vi "ADCP_Get_Parameter_Instance.vi"(8 "error in (no error)":errorcluster, 9 "Parameter Index":i32=-1, 10 "Parameter name":string, 11 "ADCP in":refnum<class "ADCP.lvclass">) -> (0 "error out":errorcluster, 1 "Data Packet":T2, 2 "Parameter":T3, 3 "ADCP out":refnum<class "ADCP.lvclass">)   [LabVIEW 2017, in "ADCP.lvclass"]
uses:
  ADCP.lvclass
  ADCP_Data_Packet_Transmit_Mode.ctl
  ADCP.lvclass/ADCP.ctl
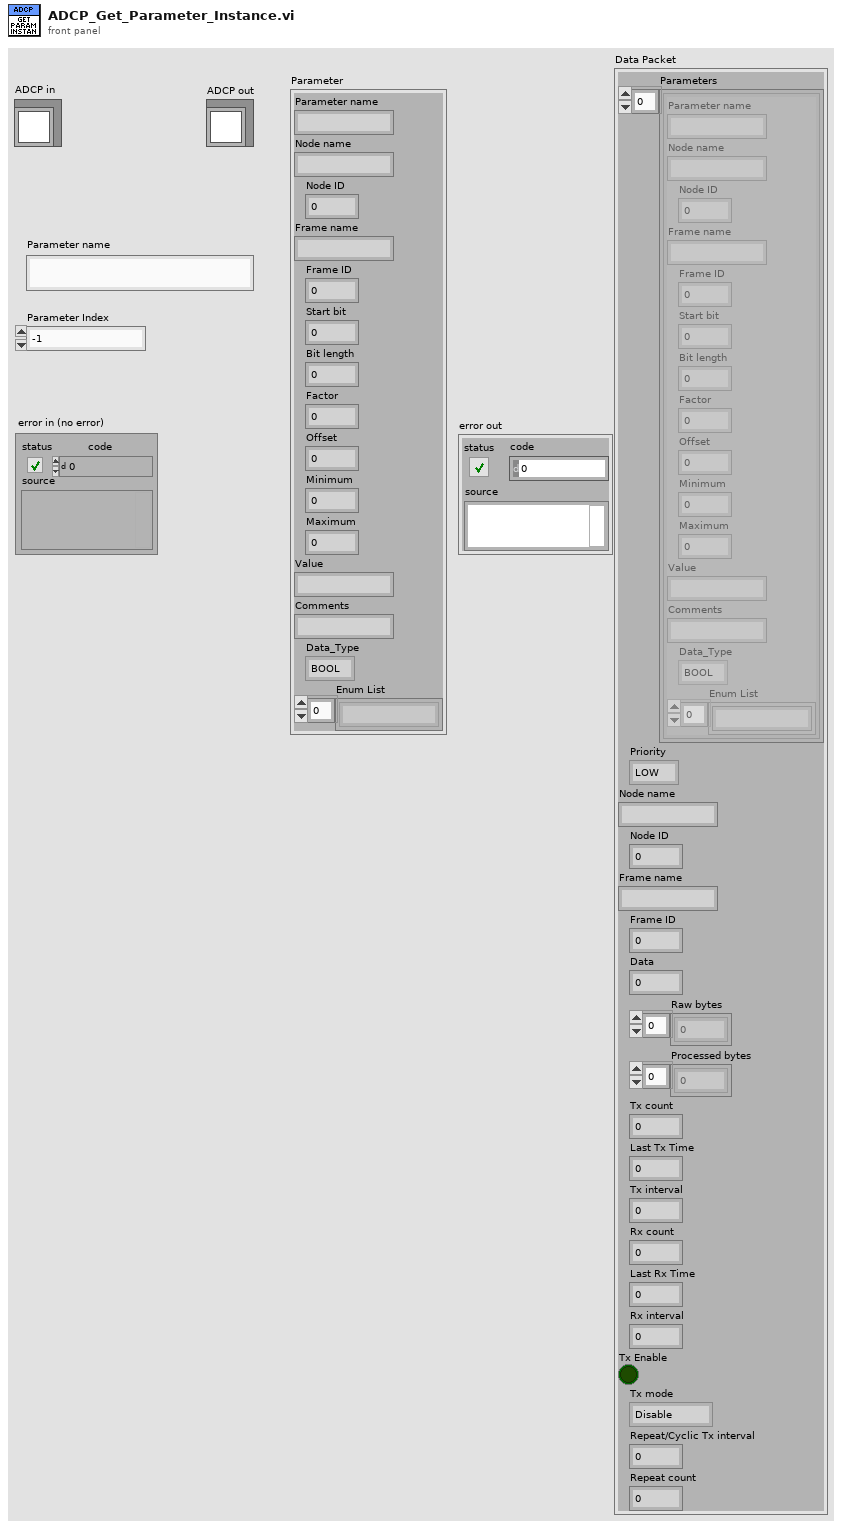
[diagram p1: front panel]
types:
  T1 = typedef "ADCP.lvclass/ADCP_Data_Packet_Transmit_Mode.ctl" = enum16{"Disable", "Single", "Cyclic", "Repeat"}
  T2 = cluster{"Parameters":cluster{"Parameter name":string, "Node name":string, "Node ID":u8, "Frame name":string, "Frame ID":u8, "Start bit":u32, "Bit length":u32, "Factor":dbl, "Offset":dbl, "Minimum":dbl, "Maximum":dbl, "Value":string, "Comments":string, "Data_Type":enum16{"BOOL", "UNSIGNED", "SIGNED", "FLOAT32", "ENUM"}, "Enum List":string[]}[], "Priority":enum16{"LOW", "HIGH"}, "Node name":string, "Node ID":u8, "Frame name":string, "Frame ID":u8, "Data":u32, "Raw bytes":u8[], "Processed bytes":u8[], "Tx count":i32, "Last Tx Time":u32, "Tx interval":u32, "Rx count":i32, "Last Rx Time":u32, "Rx interval":u32, "Tx Enable":bool, "Tx mode":T1, "Repeat/Cyclic Tx interval":u32, "Repeat count":u16}
  T3 = cluster{"Parameter name":string, "Node name":string, "Node ID":u8, "Frame name":string, "Frame ID":u8, "Start bit":u32, "Bit length":u32, "Factor":dbl, "Offset":dbl, "Minimum":dbl, "Maximum":dbl, "Value":string, "Comments":string, "Data_Type":enum16{"BOOL", "UNSIGNED", "SIGNED", "FLOAT32", "ENUM"}, "Enum List":string[]}
  T4 = cluster{"Parameter name":string, "Node name":string, "Node ID":u8, "Frame name":string, "Frame ID":u8, "Start bit":u32, "Bit length":u32, "Factor":dbl, "Offset":dbl, "Minimum":dbl, "Maximum":dbl, "Value":string, "Comments":string, "Data_Type":enum16{"BOOL", "UNSIGNED", "SIGNED", "FLOAT32", "ENUM"}, "Enum List":string[]}[]
  T5 = cluster{"Parameters":cluster{"Parameter name":string, "Node name":string, "Node ID":u8, "Frame name":string, "Frame ID":u8, "Start bit":u32, "Bit length":u32, "Factor":dbl, "Offset":dbl, "Minimum":dbl, "Maximum":dbl, "Value":string, "Comments":string, "Data_Type":enum16{"BOOL", "UNSIGNED", "SIGNED", "FLOAT32", "ENUM"}, "Enum List":string[]}[], "Priority":enum16{"LOW", "HIGH"}, "Node name":string, "Node ID":u8, "Frame name":string, "Frame ID":u8, "Data":u32, "Raw bytes":u8[], "Processed bytes":u8[], "Tx count":i32, "Last Tx Time":u32, "Tx interval":u32, "Rx count":i32, "Last Rx Time":u32, "Rx interval":u32, "Tx Enable":bool, "Tx mode":T1, "Repeat/Cyclic Tx interval":u32, "Repeat count":u16}[]
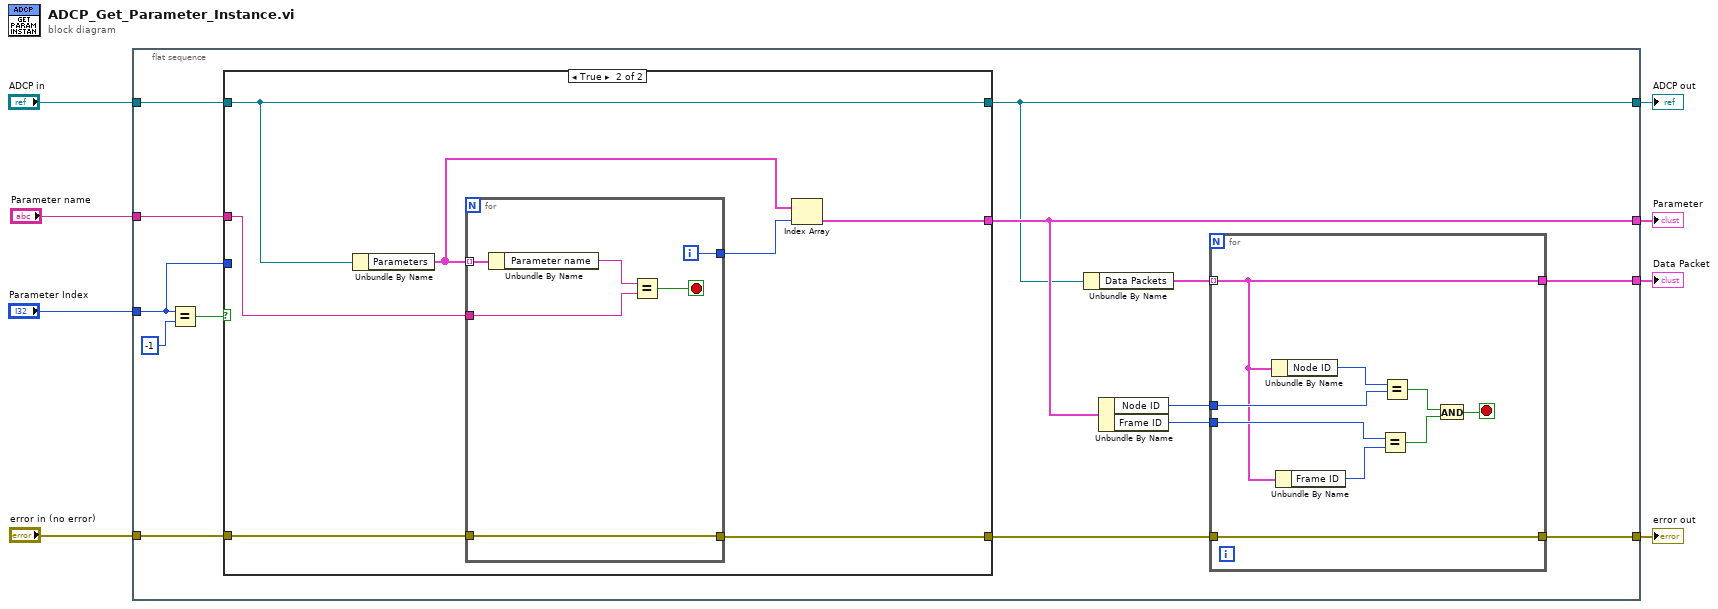
[diagram p0: block diagram]
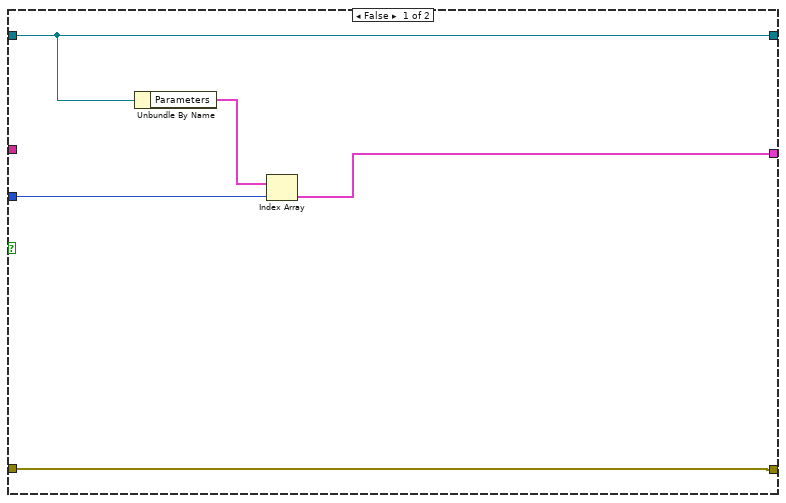
[diagram p2: hidden frame]
diagram:
  n1 = flat-sequence {
    tunnel: "ADCP in" -> [w19]
    tunnel: "Parameter name" -> [w18]
    tunnel: "Parameter Index" -> [w17]
    tunnel: "error in (no error)" -> [w22]
    tunnel: [w14] -> w4
    tunnel: [w11] -> w3
    tunnel: [w10] -> w2
    tunnel: [w9] -> w1
    frame #0 {
      n2 = Equal?(x=w17, y=-1) -> (x = y?=w21:bool)
      n3 = case shown="True" w21 {
        tunnel: w22 -> [w33 w43]
        tunnel: w19 -> [w32 w37]
        tunnel: w18 -> [_ w42]
        tunnel: w17 -> [w35 _]
        tunnel: [w34 w39] -> w14
        tunnel: [w33 w38] -> w16
        tunnel: [w32 w37] -> w9
        frame False {
          n4 = Unbundle By Name(w32) -> ("Parameters"=w36:T4)
          n5 = Index Array(array=w36, index=w35) -> (element=w34:T3)
        }
        frame True {
          n6 = Unbundle By Name(w37) -> ("Parameters"=w41:T4)
          n7 = for {
            tunnel: w41 -> [w49] mode=indexing
            tunnel: w43 -> [w45]
            tunnel: w42 -> [w47]
            tunnel: [w45] -> w38
            tunnel: [w44] -> w40
            i -> [w44]
            stop <- w46 stop-if-true
            n8 = Unbundle By Name(w49) -> ("Parameter name"=w48:string)
            n9 = Equal?(x=w48, y=w47) -> (x = y?=w46:bool)
          }
          n10 = Index Array(array=w41, index=w40) -> (element=w39:T3)
        }
      }
      n11 = Unbundle By Name(w9) -> ("Data Packets"=w15:T5)
      n12 = Unbundle By Name(w14) -> ("Node ID"=w13:u8, "Frame ID"=w12:u8)
      n13 = for {
        tunnel: w16 -> [w24]
        tunnel: w15 -> [w23] mode=indexing
        tunnel: w13 -> [w31]
        tunnel: w12 -> [w28]
        tunnel: [w24] -> w11
        tunnel: [w23] -> w10
        stop <- w25 stop-if-true
        n14 = Unbundle By Name(w23) -> ("Node ID"=w30:u8)
        n15 = Unbundle By Name(w23) -> ("Frame ID"=w29:u8)
        n16 = Equal?(x=w28, y=w29) -> (x = y?=w26:bool)
        n17 = Equal?(x=w30, y=w31) -> (x = y?=w27:bool)
        n18 = And(x=w27, y=w26) -> (x .and. y?=w25:bool)
      }
    }
  }
  "Parameter" <- w4
  "error out" <- w3
  "Data Packet" <- w2
  "ADCP out" <- w1
